vi "USB4704 #2 Buffered AI V1.vi"(6 "TimeOut":i32, 9 "Cycles":i32, 10 "Rate":i32, 11 "Start/Stop":bool) -> (0 "error out":errorcluster)   [LabVIEW 2013]
uses:
  <vilib>/Platform/TimedLoop/XDataNode/timing_clust.ctl
  <vilib>/Platform/TimedLoop/XDataNode/nitl_modes.ctl
  <vilib>/Platform/TimedLoop/XDataNode/wakeup.ctl
  <vilib>/platform/TimedLoop/XDataNode/XDataNode.xnode
  <vilib>/Platform/TimedLoop/XDataNode/XDNodeRunTimeDep.lvlib
panel:
  out "loop time":dbl
  out "Waveform Graph":dynamicdata(graph)
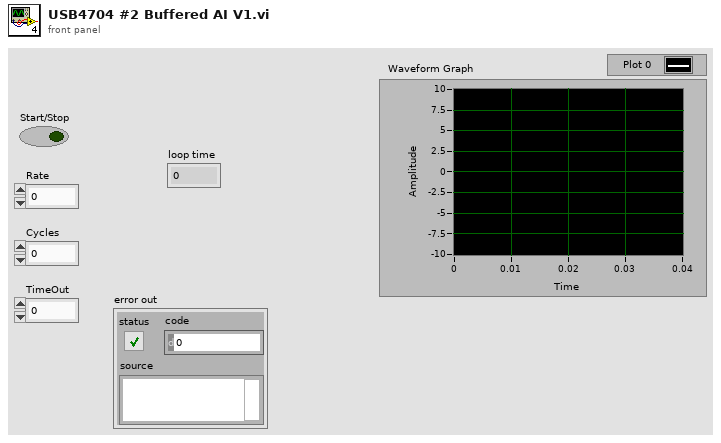
[diagram p1: front panel]
types:
  T1 = typedef "XDNodeRunTimeDep.lvlib/timing_clust.ctl" = cluster{"Expected End [f-1]":u64, "Actual End [f-1]":u64, "Finished Late? [f-1]":bool, "Expected End [i-1]":u64, "Actual End [i-1]":u64, "Finished Late? [i-1]":bool, "Expected Start [i]":u64, "Actual Start [i]":u64, "Expected Start [f]":u64, "Actual Start [f]":u64, "Source Name":string, "Structure Name":string, "Period":i64, "Deadline":i64, "Offset":i64, "Start":i64, "Priority":i32, "Timeout":i32, "Mode":T2, "Wakeup Reason":T3, "Error":errorcluster, "Source Type":string, "Secondary Source Type":string, "Global End Time":u64, "Global Start Time":u64, "Frame Duration":u64, "Iteration Duration":u64, "Assigned CPU":i32, "I/O Scan Engine Mode":u32}
  T2 = typedef "XDNodeRunTimeDep.lvlib/nitl_modes.ctl" = enum32{"No Change", "Process missed periods, maintain original phase", "Discard missed periods, maintain original phase", "Process missed periods, ignore original phase", "Discard missed periods, ignore original phase"}
  T3 = typedef "XDNodeRunTimeDep.lvlib/wakeup.ctl" = enum32{"Normal", "Aborted", "Asynchronous wakeup", "Timing source error", "Timed loop error", "Timeout"}
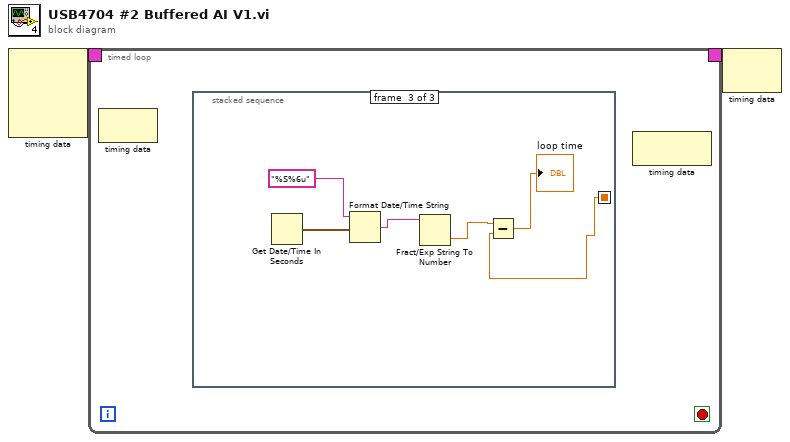
[diagram p0: block diagram]
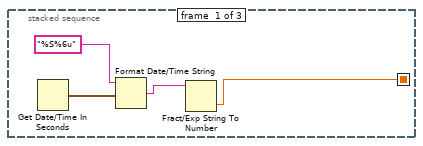
[diagram p2: hidden frame]
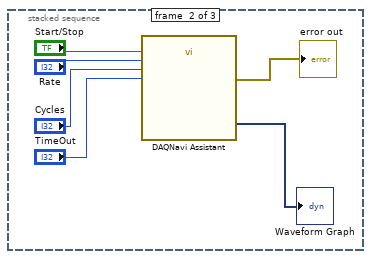
[diagram p3: hidden frame]
diagram:
  n1 = node-c288() -> (w2:T1)  [unwired: 4 in]
  n2 = timed-loop {
    timing: w2 -> [_]
    timing-out: [_] -> w1
    stop <- _ stop-if-true
    n3 = node-c288() -> ()  [unwired: 1 in, 1 out]
    n4 = stacked-sequence {
      seq-local: [w3 _ _] -> [_ _ w14]
      frame #0 {
        n5 = Get Date/Time In Seconds() -> (seconds since 1Jan1904=w5:timestamp)
        n6 = Format Date/Time String(time format string (%c)="%S%6u", seconds (now)=w5) -> (date/time string=w4:string)  [unwired: 1 in]
        n7 = Fract/Exp String To Number(string=w4) -> (number=w3:dbl)  [unwired: 3 in, 1 out]
      }
      frame #1 {
        n8 = call "DAQNavi Assistant"("stop(true)"="Start/Stop", "conversion rate(Hz)"="Rate", "samples"="Cycles", "time out(10s)"="TimeOut") -> ("error out"=→"error out":errorcluster, "data out(DDT)"=→"Waveform Graph":dynamicdata)  [unwired: 22 in]
      }
      frame #2 {
        n9 = Get Date/Time In Seconds() -> (seconds since 1Jan1904=w17:timestamp)
        n10 = Format Date/Time String(time format string (%c)="%S%6u", seconds (now)=w17) -> (date/time string=w16:string)  [unwired: 1 in]
        n11 = Fract/Exp String To Number(string=w16) -> (number=w15:dbl)  [unwired: 3 in, 1 out]
        n12 = Subtract(x=w15, y=w14) -> (x-y=→"loop time":dbl)
      }
    }
    n13 = node-c288() -> ()  [unwired: 1 in, 1 out]
  }
  n14 = node-c288(w1) -> ()  [unwired: 1 out]
